vi "libssh2_session_handshake.vi"(8 "error in (no error)":errorcluster, 10 "socket":u64, 11 "Session":T1) -> (0 "error out":errorcluster, 3 "return value":i32)   [LabVIEW 2013, in "libssh2.lvlib"]
uses:
  libssh2.lvlib
  Session Refnum.ctl
  libssh2.dll
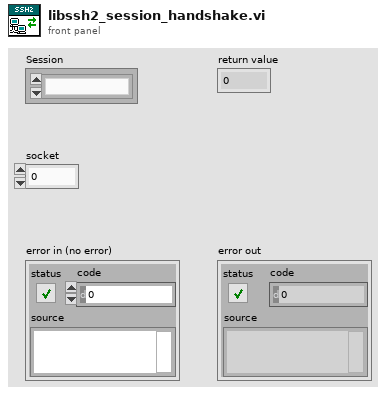
[diagram p1: front panel]
types:
  T1 = typedef "libssh2.lvlib/Session Refnum.ctl" = refnum<k1>
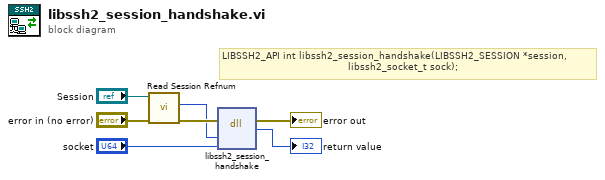
[diagram p0: block diagram]
diagram:
  # "LIBSSH2_API int libssh2_session_handshake(LIBSSH2_SESSION *session,\n                                          libssh2_socket_t sock);"
  n1 = call "Read Session Refnum.vi"("error in (no error)"="error in (no error)", "Session"="Session") -> ("error out"=w3:errorcluster, "LIBSSH2_SESSION*"=w1:u64)  [unwired: 8 in]
  n2 = dll-call lib="C:/Users/pasca/source/repos/libssh2-labview/libssh2**.*" fn="libssh2_session_handshake"(error in=w3, "session"=w1, "socket"="socket") -> (error out=→"error out":errorcluster, "return value"=→"return value":i32)  [unwired: 4 in, 1 out]
